vi "CreatePrivateEvents.vi"(8 "error in (no error)":errorcluster, 11 "Generator":refnum<class "Generator.lvclass">) -> (0 "error out":errorcluster, 3 "Generator out":refnum<class "Generator.lvclass">)   [LabVIEW 2019, in "Generator.lvclass"]
uses:
  Generator.lvclass
  typedefs/Message--Cluster.ctl
  typedefs/Sweep.Configuration--Cluster.ctl
  typedefs/Sweep.Channel--Cluster--Array.ctl
  typedefs/Sweep.Channel--Cluster.ctl
  typedefs/Sweep.Pattern--Enum.ctl
  typedefs/Sampling--Cluster.ctl
  typedefs/AO.Channel--Cluster--Array.ctl
  typedefs/AO.Channel--Cluster.ctl
  typedefs/AO.Channel.Function--Enum.ctl
  typedefs/WaveformQueues--Cluster.ctl
  Generator.lvclass/Generator.ctl
  <vilib>/JKI/JKI SMO/SMO/SMO.lvclass
  typedefs/Generator.Command--enum.ctl
  typedefs/REF.Channel--Cluster--Array.ctl
  typedefs/REF.Channel--Cluster.ctl
panel:
  # "For instructions on how to use the JKI State Machine Objects, examples and video tutorials, visit:\nhttp://jki.net/state-machine-objects/\n\nJKI State Machine Objects™\nhttp://jki.net/state-machine-objects/\nCopyright (C) 2005-2015, JKI <info@jki.net>\nALL RIGHTS RESERVED"
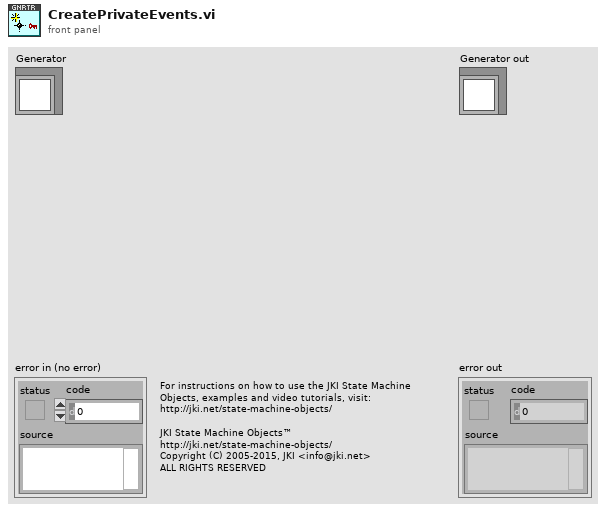
[diagram p1: front panel]
types:
  T1 = typedef "Generator.lvclass/REF.Channel--Cluster--Array.ctl" = T2[]
  T2 = typedef "Generator.lvclass/REF.Channel--Cluster.ctl" = cluster{"Enable?":bool, "Channel":i32, "Frequency":dbl, "Phase":dbl, "TC":dbl, "Roll-Off":i32}
  T3 = typedef "Generator.lvclass/Generator.Command--enum.ctl" = enum16{"start", "stop", "start sweep", "stop sweep"}
  T4 = typedef "Generator.lvclass/WaveformQueues--Cluster.ctl" = cluster{"AO":refnum<queue>, "REF_X":refnum<queue>, "REF_Y":refnum<queue>}
  T5 = typedef "Generator.lvclass/AO.Channel--Cluster--Array.ctl" = T6[]
  T6 = typedef "Generator.lvclass/AO.Channel--Cluster.ctl" = cluster{"Enable?":bool, "Channel":i32, "Amplitude":dbl, "Offset":dbl, "Frequency":dbl, "Phase":dbl, "Function":T7, "Sweeping?":bool, "Limit AC?":bool, "Limit DC?":bool, "Duty Cycle?":bool, "Duty Cycle":dbl}
  T7 = typedef "Generator.lvclass/AO.Channel.Function--Enum.ctl" = enum16{"sine", "square", "triangle", "saw"}
  T8 = typedef "Generator.lvclass/Sampling--Cluster.ctl" = cluster{"Fs":dbl, "#s":dbl}
  T9 = typedef "Generator.lvclass/Sweep.Configuration--Cluster.ctl" = cluster{"Sweep Time (s)":dbl, "Initial Wait (s)":dbl, "Return to Start":bool, "Channels":T10}
  T10 = typedef "Generator.lvclass/Sweep.Channel--Cluster--Array.ctl" = T11[]
  T11 = typedef "Generator.lvclass/Sweep.Channel--Cluster.ctl" = cluster{"Enable?":bool, "Channel":u16, "Start":dbl, "End":dbl, "Pattern":T12, "Table":dbl[]}
  T12 = typedef "Generator.lvclass/Sweep.Pattern--Enum.ctl" = enum16{"Ramp /", "Ramp /\\", "Smooth Ramp _/", "Smooth Ramp _/\\_", "Table"}
  T13 = typedef "Generator.lvclass/Message--Cluster.ctl" = cluster{"Command":string, "Data":variant}
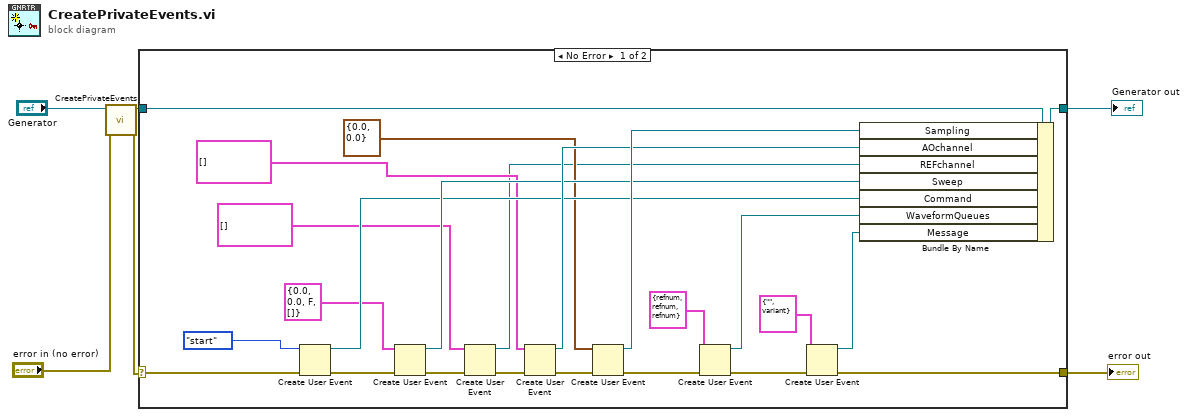
[diagram p0: block diagram]
diagram:
  n1 = call-parent "CreatePrivateEvents.vi"("error in (no error)"="error in (no error)", "SMO"="Generator") -> ("error out"=w4:errorcluster, "SMO out"=w5:refnum<class "Generator.lvclass">)  [unwired: 8 in]
  n2 = case shown="No Error" w4 {
    selector: w4 -> [w19 w32]
    tunnel: [w21 w32] -> w2
    tunnel: [w30 w31] -> w3
    tunnel: w5 -> [w29 w31]
    frame No Error {
      n3 = Create User Event(user event datatype=Generator.Command--enum."start" ("command"), error in=w19) -> (user event=w17:refnum<user-event>, error out=w18:errorcluster)
      n4 = Create User Event(user event datatype=T9 {"Sweep Time (s)"=0.0, "Initial Wait (s)"=0.0, "Return to Start"=FALSE, "Channels"=[]} ("configuration.Sweep"), error in=w18) -> (user event=w23:refnum<user-event>, error out=w27:errorcluster)
      n5 = Create User Event(user event datatype=T1 [] ("REF Channels"), error in=w27) -> (user event=w7:refnum<user-event>, error out=w26:errorcluster)
      n6 = Create User Event(user event datatype=T5 [] ("AO Channels"), error in=w26) -> (user event=w24:refnum<user-event>, error out=w28:errorcluster)
      n7 = Create User Event(user event datatype=T8 {"Fs"=0.0, "#s"=0.0} ("configuration.sampling"), error in=w28) -> (user event=w25:refnum<user-event>, error out=w13:errorcluster)
      n8 = Create User Event(user event datatype=T4 {"AO"=refnum, "REF_X"=refnum, "REF_Y"=refnum} ("WaveformQueues"), error in=w13) -> (user event=w10:refnum<user-event>, error out=w12:errorcluster)
      n9 = Create User Event(user event datatype=T13 {"Command"="", "Data"=variant} ("Message"), error in=w12) -> (user event=w22:refnum<user-event>, error out=w21:errorcluster)
      n10 = Bundle By Name(cluster=w29, "Sampling"=w25, "AOchannel"=w24, "REFchannel"=w7, "Sweep"=w23, "Command"=w17, "WaveformQueues"=w10, "Message"=w22) -> (w30:refnum<class "Generator.lvclass">)
    }
    frame Error {
    }
  }
  "error out" <- w2
  "Generator out" <- w3
